vi "AOTF signals.vi"() -> ()   [LabVIEW 2020]
uses:
  <vilib>/DAQmx/write.llb/DAQmx Write (Analog 1D Wfm NChan NSamp).vi
  <vilib>/DAQmx/create/channels.llb/DAQmx Create Channel (AO-Voltage-Basic).vi
  <vilib>/DAQmx/configure/timing.llb/DAQmx Timing (Use Waveform).vi
  <vilib>/DAQmx/miscellaneous.llb/DAQmx Fill In Error Info.vi
  <vilib>/measure/NI_MABase.lvlib
panel:
  out "LabVIEW generated Sawtooth input (blue) and Camera trigger (red)":waveform(dbl)[](graph)=[{"t0"=timestamp(0 s since 1904-01-01), "dt"=0.0009854644000985464, "Y"=array[3075 elements]}, {"t0"=timestamp(0 s since 1904-01-01), "dt"=0.0009854644000985464, "Y"=array[3075 elements]}, {"t0"=timestamp(0 s since 1904-01-01), "dt"=0.0009854644000985464, "Y"=array[3075 elements]}]
  out "# Samples written per channel 2":u32=3075
  in  "Stop 2":bool
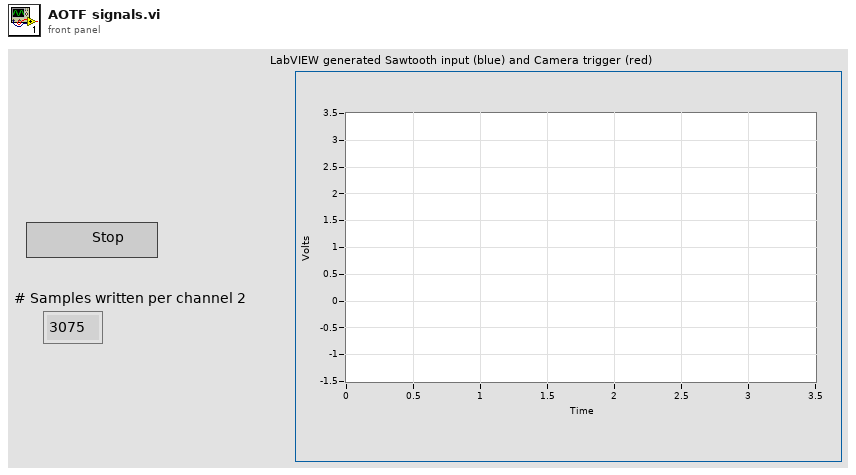
[diagram p1: front panel]
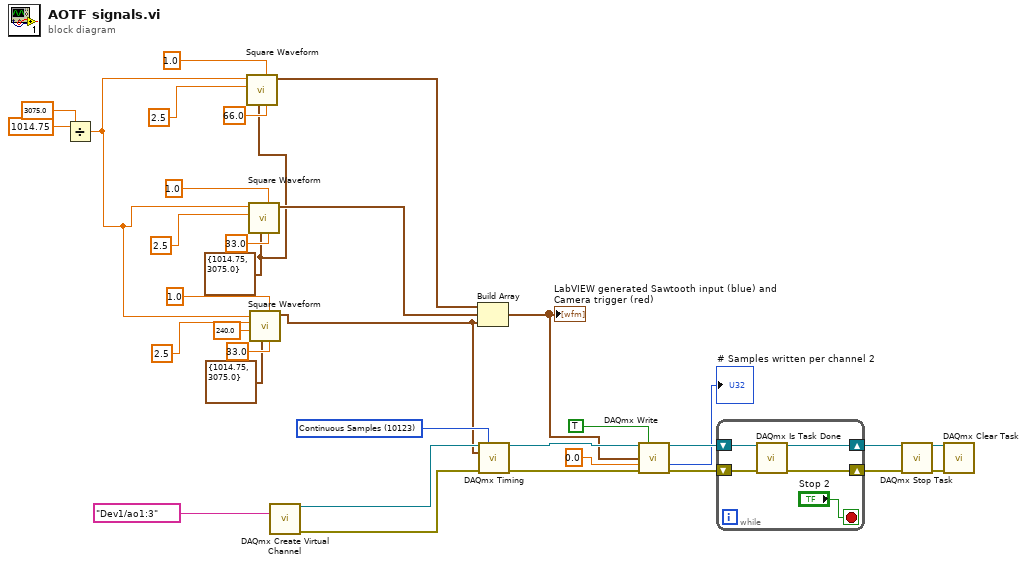
[diagram p0: block diagram]
diagram:
  w2 = cluster{"Fs":dbl, "#s":dbl} {"Fs"=1014.75, "#s"=3075.0} ("sampling info")
  w29 = 10123 items=["Finite Samples"=10178, "Continuous Samples"=10123, "Hardware Timed Single Point"=12522] ("sample mode")
  n1 = Divide(x=1014.75, y=3075.0) -> (x/y=w1:dbl)
  n2 = call <vilib>:"Square Waveform.vi"("duty cycle (%)"=66.0, "offset"=1.0, "sampling info"=w2, "amplitude"=2.5 ("Amplitude for laser 1 (Max value 2.5)"), "frequency"=w1) -> ("signal out"=w17:waveform(dbl))  [unwired: 5 in, 1 out]
  n3 = call <vilib>:"Square Waveform.vi"("duty cycle (%)"=33.0, "offset"=1.0, "sampling info"=w2, "amplitude"=2.5 ("Amplitude for laser 1 (Max value 2.5)"), "frequency"=w1) -> ("signal out"=w11:waveform(dbl))  [unwired: 5 in, 1 out]
  n4 = call <vilib>:"Square Waveform.vi"("duty cycle (%)"=33.0, "offset"=1.0, "sampling info"=cluster{"Fs":dbl, "#s":dbl} {"Fs"=1014.75, "#s"=3075.0}, "phase"=240.0, "amplitude"=2.5 ("Amplitude for laser 1 (Max value 2.5)"), "frequency"=w1) -> ("signal out"=w7:waveform(dbl))  [unwired: 4 in, 1 out]
  n5 = call-poly <vilib>:"DAQmx Create Virtual Channel.vi"("physical channels"=tag "Dev1/ao1:3") -> ("task out"=w31:refnum<k21>, "error out"=w30:errorcluster)  [unwired: 13 in]
  n6 = Build Array(w17, w11, w7) -> (w18:waveform(dbl)[])
  "LabVIEW generated Sawtooth input (blue) and Camera trigger (red)" <- w18
  n7 = call-poly <vilib>:"DAQmx Timing.vi"("task/channels in"=w31, "sample mode"=w29, "waveform"=w7, "error in"=w30) -> ("task out"=w26:refnum<k21>, "error out"=w25:errorcluster)  [unwired: 10 in]
  n8 = call-poly <vilib>:"DAQmx Write.vi"("task/channels in"=w26, "auto start"=TRUE, "data"=w18, "timeout"=0.0, "error in"=w25) -> ("task out"=w27:refnum<k21>, "number of samples written per channel"=→"# Samples written per channel 2":u32, "error out"=w28:errorcluster)  [unwired: 8 in]
  n9 = while {
    shift-right: [w36] -> w23
    shift-left: w27 -> [w39]
    shift-right: [w37] -> w24
    shift-left: w28 -> [w38]
    stop <- "Stop 2" stop-if-true
    n10 = call <vilib>:"DAQmx Is Task Done.vi"("task/channels in"=w39, "error in"=w38) -> ("task out"=w36:refnum<k21>, "error out"=w37:errorcluster)  [unwired: 11 in, 1 out]
  }
  n11 = call <vilib>:"DAQmx Stop Task.vi"("task/channels in"=w23, "error in"=w24) -> ("task out"=w32:refnum<k21>, "error out"=w33:errorcluster)  [unwired: 12 in]
  n12 = call <vilib>:"DAQmx Clear Task.vi"("task in"=w32, "error in"=w33) -> ()  [unwired: 13 in, 1 out]
